vi "ABR3-Set Level.vi"(0 "Runtime":T26={"Ceiling"=0.0, "Threshold"=0.0, "Crossed?"=FALSE, "Step"=0, "Stop"=0, "Avgs"=0, "Level"=0.0, "AI Npts"=0, "Doubled?"=FALSE, "Gain"=0.0, "NWindowPts"=0, "dt"=0.0, "Cal"=path "", "Freq"=0.0, "AO Channels"=[], "AltPol"=FALSE, "AO Npts"=0, "AO Fs"=0.0, "Start"=0, "Stop max"=0, "Ear"=enum."Right", "Waveform"=enum."TONE PIP", "RepRate"=0.0, "CAP or ABR"=1, "LMasker"=0.0, "SeqVar"=enum."Signal Level", "Reps/buffer"=0, "Avg Mode"=enum."Neural/CM", "Wav"=path "", "Order"=enum."Sequential", "Levels"=[], "ControlVal"=0.0, "innerIndex"=0, "indexStep"=0} {"CAP or ABR" items=["CAP", "ABR"]}, 5 "StimChans":T1[](xcontrol), 11 "error in (no error)":errorcluster) -> (6 "StimChans out":T1[](xcontrol), 13 "Level":dbl, 15 "error out":errorcluster)   [LabVIEW 2020]
uses:
  TypeDefs/ABR3-Runtime Data.ctl
  epl-vi-lib/Utility VIs/Type Defs/Left-Right ring.ctl
  TypeDefs/ABR-Waveform Enum.ctl
  TypeDefs/ABR3-Seq Var Enum.ctl
  epl-vi-lib/Signal Synthesis VIs/Controls/Multichannel (Full)/Multichannel (Full).xctl
  epl-vi-lib/Signal Synthesis VIs/Controls/Waveform XCtl/Waveform Enum.ctl
  epl-vi-lib/Signal Synthesis VIs/Top Level VIs/Stimulus-Set Level (full wrapper).vi
  epl-vi-lib/Utility VIs/Math VIs/dB to Linear (scalar).vi
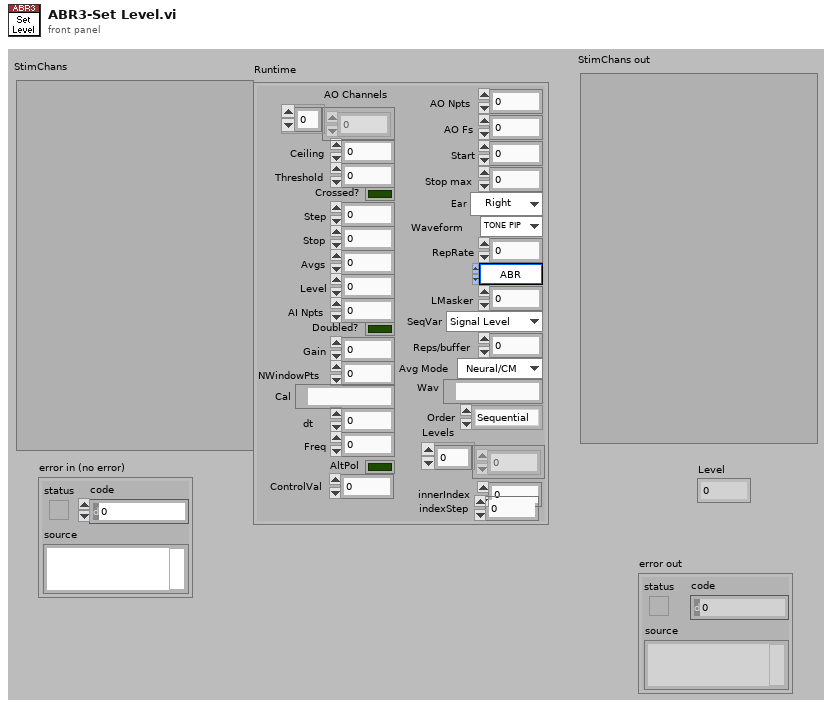
[diagram p1: front panel]
types:
  T1 = typedef "Stimulus Channel (Full).xctl/Full Stimulus Channel Data.ctl" = cluster{"Waveform":T2, "Filter":T19, "Burst":T21, "Level":T22, "Name":string, "Advanced":T24, "SAM":T25}
  T2 = typedef "Waveform XCtl.xctl/Waveform Data.ctl" = cluster{"Type":T3, "Tone":T4, "Pulse Train":T5, "Noise":T8, "File":T9, "FMSweep":T10, "Chirp Train":T11, "Complex Tone":cluster{"Params":T13, "Data":T15}, "Moving Ripple":T16}
  T3 = typedef "Waveform Enum.ctl" = enum16{"OFF", "Tone", "Noise", "Pulse Train", "File", "FM Sweep", "Chirp Train", "Complex Tone", "FM Tone", "Moving Ripple"}
  T4 = typedef "Tone Params.ctl" = cluster{"Frequency (kHz)":dbl, "Last Freq":dbl, "Last Phase":dbl}
  T5 = typedef "Pulse Train Params.ctl" = cluster{"Pulse width (us)":dbl, "Pulse rate (Hz)":dbl, "Gap (ms)":dbl, "Polarity":T6, "PT State":T7, "Asynch":bool}
  T6 = typedef "Pulse Polarity.ctl" = enum16{"POS", "NEG", "POS-NEG", "NEG-POS"}
  T7 = typedef "PT-Continuous State.ctl" = cluster{"Template":dbl[], "Nperiod":i32, "Index":i32, "Pulse Rate (Hz)":dbl, "Phase (cycles)":dbl, "Noff":i32}
  T8 = typedef "Noise Params.ctl" = cluster{"InvFilt":bool, "Noise":dbl[], "CurPt":i32, "Aweight":bool, "Seed":i32, "afile":path}
  T9 = typedef "StimFile-Params.ctl" = cluster{"Filename":path, "Signal":dbl[], "Channel":i32, "stream":bool, "offset":i32, "nreps":i32, "loops":i32, "Randomize":bool, "order":i32[], "Seed":i32, "Tokens":i32}
  T10 = typedef "FM Sweep Params.ctl" = cluster{"Rate (oct/s)":dbl, "Fmin (Hz)":dbl, "Fmax (Hz)":dbl, "Ramp (ms)":dbl, "Linear":bool}
  T11 = typedef "Chirp Train.ctl" = cluster{"Params":T12, "Data":cluster{"WF":dbl[]}}
  T12 = typedef "Chirp Train Params.ctl" = cluster{"Fmin (kHz)":dbl, "Fmax (kHz)":dbl, "Compensate":bool, "Duration (ms)":dbl}
  T13 = typedef "CT-Params.ctl" = cluster{"F0 (Hz)":dbl, "Band":cluster{"Flow (Hz)":dbl, "Fhigh (Hz)":dbl}, "Phase":T14, "Min F0 (Hz)":dbl, "Max F0 (Hz)":dbl, "ContinRandPhase":bool, "Max peak factor":dbl, "Max mod depth":dbl, "MinHarmNum":i32, "MaxHarmNum":i32, "Level Mode":enum16{"per component", "overall rms"}, "% jitter":dbl}
  T14 = typedef "CT-Phase Enum.ctl" = enum16{"Cosine", "Random", "Alternating"}
  T15 = typedef "CT-Runtime Data.ctl" = cluster{"Ncomp":i32, "MinHarm":i32, "Phase":dbl[], "Amplitude":dbl[], "Npts/frame":i32, "Last F0":dbl, "Fmin":dbl, "Fmax":dbl, "Lslope":dbl, "randphase":bool, "overall rms":bool, "fmult":dbl[], "jittered":bool}
  T16 = typedef "Moving Ripple.ctl" = cluster{"Params":T17, "Data":T18}
  T17 = typedef "Moving Ripple.Params.ctl" = cluster{"Fmin":dbl, "Fmax":dbl, "Density":dbl, "Velocity":dbl, "Depth":dbl, "Phase":dbl, "Comp/oct":i32}
  T18 = typedef "Moving Ripple.Data.ctl" = cluster{"Freq":dbl[], "A":dbl[], "phase":dbl[], "Phase":dbl}
  T19 = typedef "Advanced Filter XCtl.xctl/Filter Data.ctl" = cluster{"Type":enum16{"Lowpass", "Highpass", "Bandpass", "Bandstop", "OFF"}, "CF (kHz)":dbl, "BW (kHz)":dbl, "Cascade":bool, "Quadrature":bool, "Scale Factor":dbl, "Stages":cluster{"IIR Filter":cluster{"filter structure":enum32{"IIR 2nd Order", "IIR 4th Order"}, "Reverse Coefficients":dbl[], "Forward Coefficients":dbl[]}, "State":dbl[]}[], "Class":enum16{"Elliptic", "Butterworth"}, "Order":i32, "BWUnits":T20}
  T20 = typedef "Filter-Bandwidth Units.ctl" = enum16{"Linear", "Octaves", "Min-Max"}
  T21 = typedef "Burst Control.xctl/Burst Data.ctl" = cluster{"Active":bool, "Delay (ms)":dbl, "Duration (ms)":dbl, "Ramp (ms)":dbl, "Rate (Hz)":dbl, "Trepeat (ms)":dbl, "Repeat":bool}
  T22 = typedef "Level XCtl.xctl/Level Data.ctl" = cluster{"Level":dbl, "Units":T23, "Max":dbl, "Multiplier":dbl, "Cal File":path, "Cal":cluster{"Freq (Hz)":dbl[], "Mag (dB SPL)":dbl[], "Phase (deg)":dbl[]}}
  T23 = typedef "Level Units.ctl" = enum16{"dB atten", "dB SPL", "dB re 1 Vrms", "dB V/Hz½", "mW", "dB HL", "Volts", "dB mW"}
  T24 = typedef "Advanced Stimulus Options.xctl/Advanced Stimulus Options.ctl" = cluster{"Rep Mask":string, "AltPol":bool, "Var":string, "Expr":string, "Persist":bool}
  T25 = typedef "SAM Params.ctl" = cluster{"Active":bool, "Frequency (Hz)":dbl, "Depth":dbl, "Init Phase (cycles)":dbl, "phase (degrees)":dbl, "Asynch":bool}
  T26 = typedef "ABR3-Runtime Data.ctl" = cluster{"Ceiling":dbl, "Threshold":dbl, "Crossed?":bool, "Step":i32, "Stop":i32, "Avgs":i32, "Level":dbl, "AI Npts":i32, "Doubled?":bool, "Gain":dbl, "NWindowPts":i32, "dt":dbl, "Cal":path, "Freq":dbl, "AO Channels":i32[], "AltPol":bool, "AO Npts":i32, "AO Fs":dbl, "Start":i32, "Stop max":i32, "Ear":T27, "Waveform":T28, "RepRate":dbl, "CAP or ABR":u16, "LMasker":dbl, "SeqVar":T29, "Reps/buffer":i32, "Avg Mode":enum16{"Neural/CM", "ANOW"}, "Wav":path, "Order":enum16{"Sequential", "Random"}, "Levels":dbl[], "ControlVal":dbl, "innerIndex":i32, "indexStep":i32}
  T27 = typedef "Left-Right ring.ctl" = enum16{"Right", "Left"}
  T28 = typedef "ABR-Waveform Enum.ctl" = enum16{"TONE PIP", "CLICK", "FILE", "CHIRP", "NOISE", "VERHULST"}
  T29 = typedef "ABR3-Seq Var Enum.ctl" = enum16{"Signal Level", "Masker Level"}
  T30 = enum16{"Init", "Write", "Read", "Latch setup", "Compute comp.", "Read 1 Channel"}
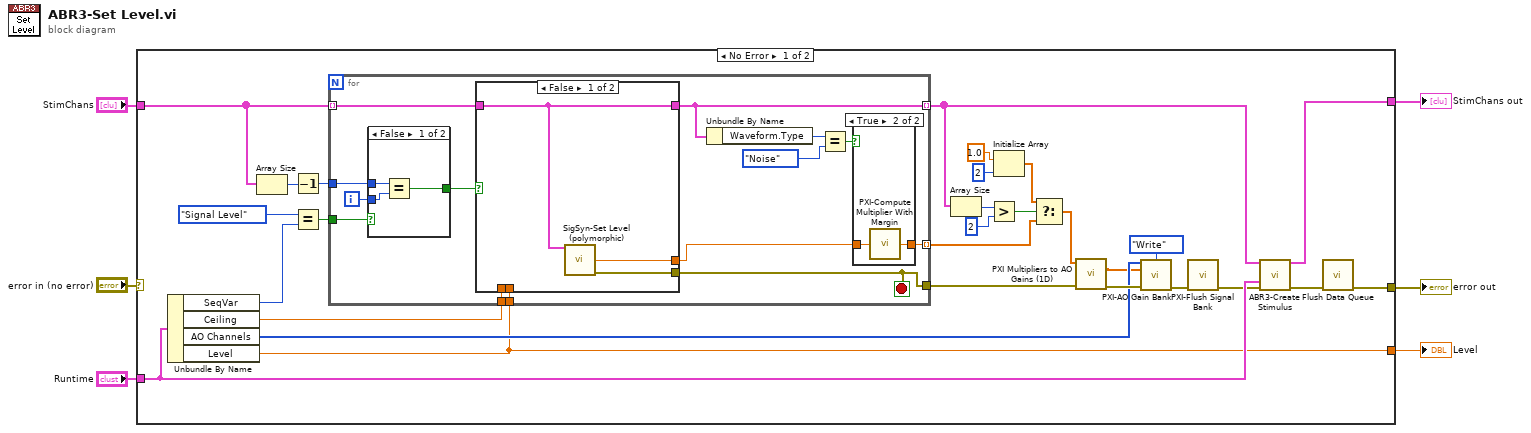
[diagram p0: block diagram]
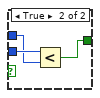
[diagram p3: hidden frame]
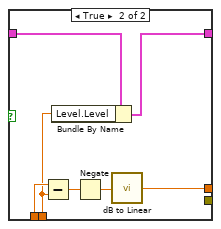
[diagram p4: hidden frame]
diagram:
  n1 = case shown="No Error" "error in (no error)" {
    selector: "error in (no error)" -> [_ w68]
    tunnel: "Runtime" -> [w29 _]
    tunnel: [w25 w68] -> w4
    tunnel: [w27 _] -> w3
    tunnel: "StimChans" -> [w21 _]
    tunnel: [w28 _] -> w1
    frame No Error {
      n2 = Unbundle By Name(w29) -> ("SeqVar"=w20:T29, "Ceiling"=w34:dbl, "AO Channels"=w32:i32[], "Level"=w27:dbl)
      n3 = Array Size(array=w21) -> (size(s)=w17:i32)
      n4 = Decrement(x=w17) -> (x-1=w16:i32)
      n5 = Equal?(x=ABR3-Seq_Var_Enum."Signal Level", y=w20) -> (x = y?=w18:bool)
      n6 = for {
        tunnel: w34 -> [w48]
        tunnel: [w40] -> w15 mode=indexing
        tunnel: w27 -> [w47]
        tunnel: [w45] -> w22
        tunnel: [w37] -> w8 mode=indexing
        tunnel: w21 -> [w46] mode=indexing
        tunnel: w18 -> [w44]
        tunnel: w16 -> [w43]
        i -> [w42]
        stop <- w45 stop-if-true
        n7 = case shown="False" w44 {
          tunnel: w43 -> [w54 w56]
          tunnel: w42 -> [w53 w57]
          tunnel: [w52 w55] -> w41
          frame False {
            n8 = Equal?(x=w54, y=w53) -> (x = y?=w52:bool)
          }
          frame True {
            n9 = Less?(x=w57, y=w56) -> (x < y?=w55:bool)
          }
        }
        n10 = case shown="False" w41 {
          tunnel: w48 -> [_ w67]
          tunnel: w47 -> [_ w66]
          tunnel: w46 -> [w58 w63]
          tunnel: [w58 w62] -> w40
          tunnel: [w60 w61] -> w36
          tunnel: [w59 _] -> w45
          frame False {
            n11 = call-poly "SigSyn-Set Level (polymorphic).vi"("Stimulus Channel"=w58) -> ("Multiplier"=w60:dbl, "error out"=w59:errorcluster)  [unwired: 10 in, 3 out]
          }
          frame True {
            n12 = Subtract(x=w67, y=w66) -> (x-y=w65:dbl)
            n13 = Bundle By Name(cluster=w63, "Level.Level"=w66) -> (w62:T1)
            n14 = Negate(x=w65) -> (-x=w64:dbl)
            n15 = call-poly "dB to Linear.vi"("dB"=w64) -> ("linear"=w61:dbl)
          }
        }
        n16 = Unbundle By Name(w40) -> ("Waveform.Type"=w39:T3)
        n17 = Equal?(x=w39, y=Waveform_Enum."Noise") -> (x = y?=w35:bool)
        n18 = case shown="True" w35 {
          tunnel: [w49 w50] -> w37
          tunnel: w36 -> [w49 w51]
          frame False {
          }
          frame True {
            n19 = call "PXI-Compute Multiplier With Margin.vi"("Mult In"=w51) -> ("Mult Out"=w50:dbl)  [unwired: 14 in]
          }
        }
      }
      n20 = Array Size(array=w15) -> (size(s)=w14:i32)
      n21 = Greater?(x=w14, y=2) -> (0:w10:bool)
      n22 = Initialize Array(1.0, 2 ("dimension size")) -> (w9:dbl[])
      n23 = Select(t=w9, s=w10, f=w8) -> (s? t:f=w7:dbl[])
      n24 = call "PXI Multipliers to AO Gains (1D).vi"("Multipliers in"=w7, "error in (no error)"=w22) -> ("Gains"=w31:dbl[], "error out"=w33:errorcluster)  [unwired: 11 in, 1 out]
      n25 = call "PXI-AO Gain Bank.vi"("AO Channels"=w32, "Action"=T30."Write", "Gains"=w31, "error in (no error)"=w33) -> ("error out"=w24:errorcluster)  [unwired: 6 in, 5 out]
      n26 = call "PXI-Flush Signal Bank.vi"("error in (no error)"=w24) -> ("error out"=w23:errorcluster)  [unwired: 10 in]
      n27 = call "ABR3-Create Stimulus.vi"("StimChans"=w15, "Runtime"=w29, "error in (no error)"=w23) -> ("StimChans out"=w28:T1[], "error out"=w26:errorcluster)  [unwired: 10 in, 1 out]
      n28 = call "Flush Data Queue.vi"("error in (no error)"=w26) -> ("error out"=w25:errorcluster)  [unwired: 10 in]
    }
    frame Error {
    }
  }
  "error out" <- w4
  "Level" <- w3
  "StimChans out" <- w1
